vi "testDLLCall.vi"() -> ()   [LabVIEW 2010]
uses:
  DLL-s/test/Debug/test.dll
panel:
  out "return type":i32
  out "arg1":i32[](array[numeric])
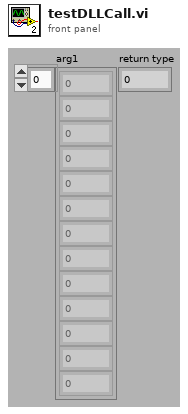
[diagram p1: front panel]
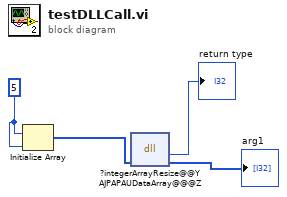
[diagram p0: block diagram]
diagram:
  w3 = 5
  n1 = Initialize Array(w3, w3) -> (w2:i32[])
  n2 = dll-call lib="D:/Liakh Tanya/Dissertation/Complex/DLL-s/test/Debug/test.dll" fn="?integerArrayResize@@YAJPAPAUDataArray@@@Z"("arg1"=w2) -> ("return type"=→"return type":i32, "arg1"=→"arg1":i32[])  [unwired: 3 in, 2 out]
